vi "Reply Timeout.vi"() -> (0 "Reply Timeout":i32)   [LabVIEW 2020, in "SECS Scenarios.lvlib" / "Scenarios Class.lvclass"]
uses:
  Scenarios Class.lvclass
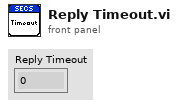
[diagram p1: front panel]
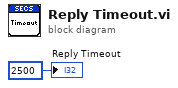
[diagram p0: block diagram]
diagram:
  "Reply Timeout" <- 2500 ("Reply Timeout")
